vi "Setup_Constants.vi"(3 "error in (no error)":errorcluster, 4 "Config In":T1={"IntTime"=100, "Samples"=3, "PowerMin"=300.0, "KneeMin"=-20.0, "KneeMax"=20.0, "Background Wl"=275.0, "Settle Delay,ms"=275, "StationId"=0.0} {"Background Wl" min=220.0 max=320.0; "IntTime" min=1 max=100000; "Samples" min=1 max=10; "PowerMin" min=0.0 max=10000.0; "KneeMin" min=-40.0 max=0.0; "KneeMax" min=0.0 max=40.0}, 5 "Instruments in":refnum<class "Instruments.lvclass">) -> (0 "error out":errorcluster, 2 "Instruments out":refnum<class "Instruments.lvclass">)   [LabVIEW 2012, in "Instruments.lvclass"]
uses:
  Instruments.lvclass
  Controls/Config.ctl
  Instruments.lvclass/Instruments.ctl
panel:
  # "Measurement Settings"
  # "Test Criteria"
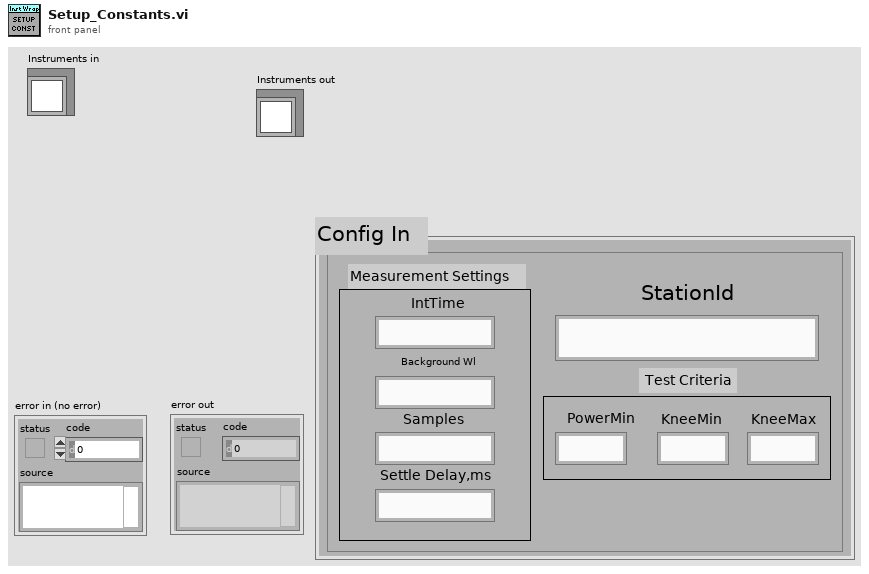
[diagram p1: front panel]
types:
  T1 = typedef "Config.ctl" = cluster{"IntTime":i32, "Samples":i32, "PowerMin":dbl, "KneeMin":dbl, "KneeMax":dbl, "Background Wl":dbl, "Settle Delay,ms":u32, "StationId":sgl}
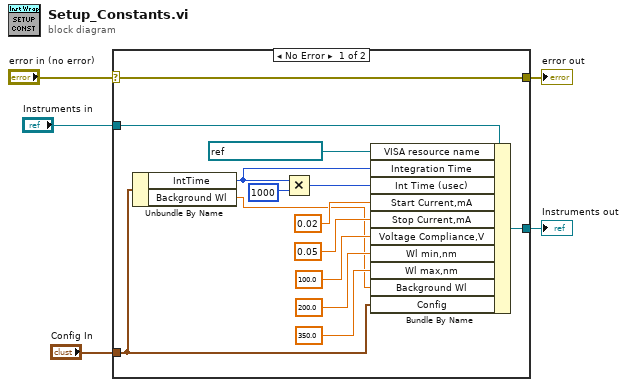
[diagram p0: block diagram]
diagram:
  n1 = case shown="No Error" "error in (no error)" {
    selector: "error in (no error)" -> [w19 w21]
    tunnel: [w19 w21] -> w4
    tunnel: [w12 w20] -> w2
    tunnel: "Instruments in" -> [w18 w20]
    tunnel: "Config In" -> [w8 _]
    frame No Error {
      n2 = Unbundle By Name(w8) -> ("IntTime"=w9:i32, "Background Wl"=w7:dbl)
      n3 = Multiply(x=w9, y=1000) -> (x*y=w10:i32)
      n4 = Bundle By Name(cluster=w18, "VISA resource name"=refnum<visa-resource-name> "GPIB0::24::INSTR" ("INSTR_PARAM.Keithley_Param.VISA resource name"), "Integration Time"=w9, "Int Time (usec)"=w10, "Start Current,mA"=0.02 ("INSTR_PARAM.Keithley_Param.Start Current,mA"), "Stop Current,mA"=0.05 ("INSTR_PARAM.Keithley_Param.Stop Current,mA"), "Voltage Compliance,V"=100.0 ("INSTR_PARAM.Keithley_Param.Voltage Compliance,V"), "Wl min,nm"=200.0 ("INSTR_PARAM.USB4000_Param.Wl min,nm"), "Wl max,nm"=350.0 ("INSTR_PARAM.USB4000_Param.Wl max,nm"), "Background Wl"=w7, "Config"=w8) -> (w12:refnum<class "Instruments.lvclass">)
    }
    frame Error {
    }
  }
  "error out" <- w4
  "Instruments out" <- w2
